vi "Register for Events.vi"(8 "error in (no error)":errorcluster, 11 "Storage in":refnum<class "Storage.lvclass">) -> (0 "error out":errorcluster, 2 "Event Registration Refnum":variant, 3 "Storage out":refnum<class "Storage.lvclass">)   [LabVIEW 2015, in "AMS UI.lvlib" / "Storage.lvclass"]
uses:
  Storage.lvclass
  eActor/eActor.lvclass/eActor.ctl
  Storage.lvclass/Storage.ctl
  eActor/eActor.lvclass
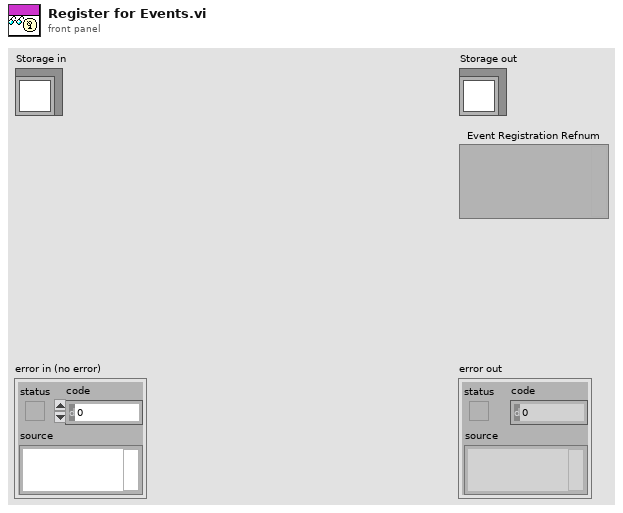
[diagram p1: front panel]
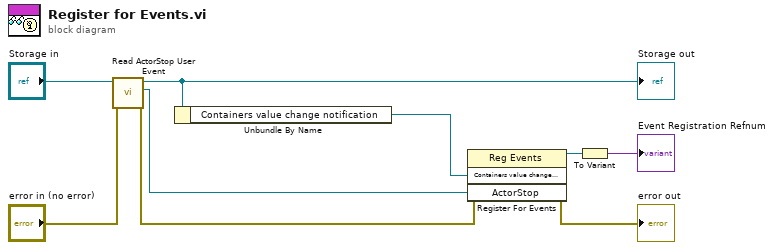
[diagram p0: block diagram]
diagram:
  n1 = call "Read ActorStop User Event.vi"("error in (no error)"="error in (no error)", "eActor in"="Storage in") -> ("error out"=w5:errorcluster, "ActorStop"=w6:refnum<user-event>, "eActor out"=w7:refnum<class "Storage.lvclass">)  [unwired: 7 in]
  "Storage out" <- w7
  n2 = Unbundle By Name(w7) -> ("Containers value change notification"=w1:refnum<user-event>)
  n3 = register-events(error in=w5, w1, w6) -> (reference out=w3:refnum<event-registration>, error out=→"error out":errorcluster)  [unwired: 1 in]
  n4 = To Variant(anything=w3) -> (Variant=→"Event Registration Refnum":variant)
